vi "FilterCANFrames.vi"(11 "remaining elements in":T1[](array[typedef]) {"type" items=["CAN Data", "CAN Remote"]; "identifier" format="%.0x"}) -> (3 "duplicates removed":T1[](array[typedef]) {"type" items=["CAN Data", "CAN Remote"]; "identifier" format="%.0x"})   [LabVIEW 2016, in "DSI-RT.lvlib"]
uses:
  DSI-RT.lvlib
  <vilib>/RioEmbeddedCAN/RioEmbeddedCAN.llb/CANFrameControl.ctl
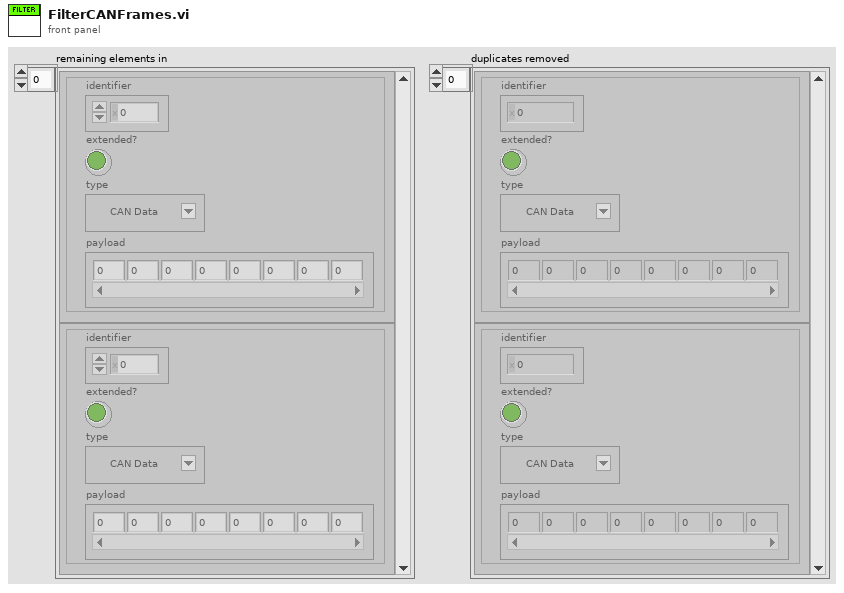
[diagram p1: front panel]
types:
  T1 = typedef "CANFrameControl.ctl" = cluster{"identifier":u32, "extended?":bool, "type":u8, "payload":u8[]}
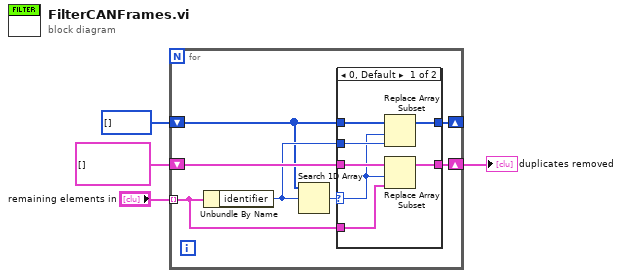
[diagram p0: block diagram]
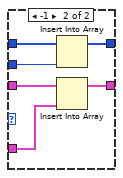
[diagram p2: hidden frame]
diagram:
  n1 = for {
    shift-right: [w11] -> w2
    shift-left: T1[] [] ("Array") -> [w10]
    tunnel: "remaining elements in" -> [w8] mode=indexing
    shift-right: [w6] -> _
    shift-left: u32[] [] -> [w5]
    n2 = Unbundle By Name(w8) -> ("identifier"=w7:u32)
    n3 = Search 1D Array(1D array=w5, element=w7) -> (index of element=w9:i32)  [unwired: 1 in]
    n4 = case shown="0, Default" w9 {
      selector: w9 -> [w13 _]
      tunnel: [w18 w23] -> w11
      tunnel: w10 -> [w17 w24]
      tunnel: w8 -> [w16 w22]
      tunnel: w7 -> [w15 w19]
      tunnel: [w14 w20] -> w6
      tunnel: w5 -> [w12 w21]
      frame 0, Default {
        n5 = Replace Array Subset(array=w12, new element=w15, index=w13) -> (w14:u32[])
        n6 = Replace Array Subset(array=w17, new element=w16, index=w13) -> (w18:T1[])
      }
      frame -1 {
        n7 = Insert Into Array(array=w21, new element=w19) -> (w20:u32[])  [unwired: 1 in]
        n8 = Insert Into Array(array=w24, new element=w22) -> (w23:T1[])  [unwired: 1 in]
      }
    }
  }
  "duplicates removed" <- w2
